vi "Temp M2 FPGA.vi"() -> ()   [LabVIEW 2011]
uses:
  <vilib>/rvi/eio/common/nirviEmuTemplateMethod_errors.vi
  <vilib>/eio/EIONode/EIONode.xnode
panel:
  in  "stop":bool
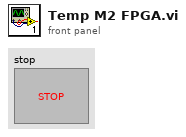
[diagram p1: front panel]
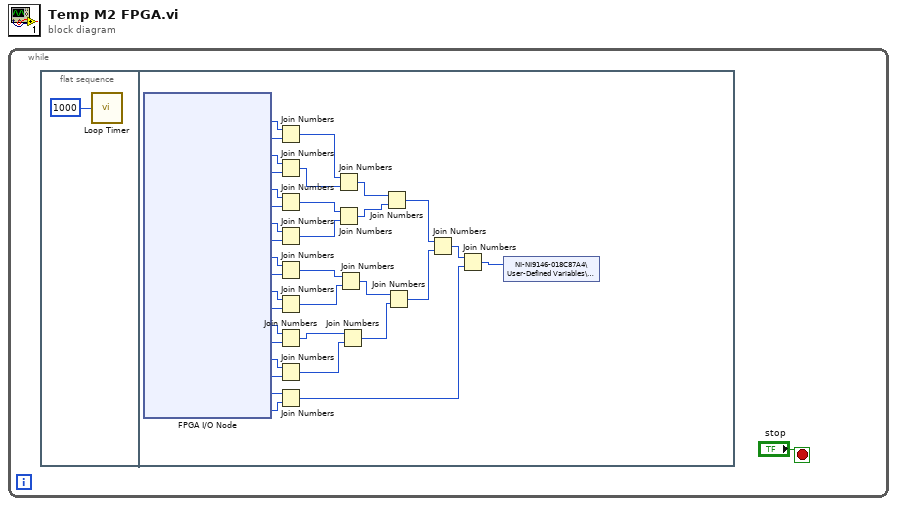
[diagram p0: block diagram]
diagram:
  n1 = while {
    stop <- "stop" stop-if-true
    n2 = flat-sequence {
      frame #0 {
        n3 = call "Loop Timer"("Count(mSec)"=u32 1000) -> ()  [unwired: 1 out]
      }
      frame #1 {
        n4 = xnode "FPGA I/O Node"() -> ("Mod1/Autozero"=w37:i32, "Mod1/CJC"=w36:i32, "Mod1/TC0"=w35:i32, "Mod1/TC1"=w34:i32, "Mod1/TC2"=w33:i32, "Mod1/TC3"=w32:i32, "Mod1/TC4"=w30:i32, "Mod1/TC5"=w29:i32, "Mod1/TC6"=w28:i32, "Mod1/TC7"=w27:i32, "Mod1/TC8"=w26:i32, "Mod1/TC9"=w31:i32, "Mod1/TC10"=w25:i32, "Mod1/TC11"=w24:i32, "Mod1/TC12"=w23:i32, "Mod1/TC13"=w22:i32, "Mod1/TC14"=w21:i32, "Mod1/TC15"=w20:i32)  [unwired: 18 in, 18 out]
        n5 = Join Numbers(hi=w37, lo=w36) -> ((hi.lo)=w19:u64)
        n6 = Join Numbers(hi=w35, lo=w34) -> ((hi.lo)=w18:u64)
        n7 = Join Numbers(hi=w33, lo=w32) -> ((hi.lo)=w17:u64)
        n8 = Join Numbers(hi=w30, lo=w29) -> ((hi.lo)=w16:u64)
        n9 = Join Numbers(hi=w28, lo=w27) -> ((hi.lo)=w15:u64)
        n10 = Join Numbers(hi=w26, lo=w31) -> ((hi.lo)=w14:u64)
        n11 = Join Numbers(hi=w25, lo=w24) -> ((hi.lo)=w13:u64)
        n12 = Join Numbers(hi=w23, lo=w22) -> ((hi.lo)=w12:u64)
        n13 = Join Numbers(hi=w21, lo=w20) -> ((hi.lo)=w4:u64)
        n14 = Join Numbers(hi=w19, lo=w18) -> ((hi.lo)=w11:u64)
        n15 = Join Numbers(hi=w17, lo=w16) -> ((hi.lo)=w10:u64)
        n16 = Join Numbers(hi=w15, lo=w14) -> ((hi.lo)=w9:u64)
        n17 = Join Numbers(hi=w13, lo=w12) -> ((hi.lo)=w8:u64)
        n18 = Join Numbers(hi=w11, lo=w10) -> ((hi.lo)=w7:u64)
        n19 = Join Numbers(hi=w9, lo=w8) -> ((hi.lo)=w6:u64)
        n20 = Join Numbers(hi=w7, lo=w6) -> ((hi.lo)=w5:u64)
        n21 = Join Numbers(hi=w5, lo=w4) -> ((hi.lo)=w3:u64)
        n22 = shared-variable "NI-NI9146-018C87A4\\User-Defined Variables\\Temp M2"(w3) -> ()  [unwired: 1 in, 1 out]
      }
    }
  }
